vi "Item Click.vi"(4 "Menu in":refnum<class "MGI_ToolStrip.lvclass">, 5 "Event Data":cluster{"sender":refnum<k24>, "e":refnum<k24>}, 6 "Control Ref":refnum<k24>, 7 "Event Common Data":T1) -> ()   [LabVIEW 2019, in "MGI_ToolStrip.lvclass"]
uses:
  MGI_ToolStrip.lvclass
  System.Windows.Forms
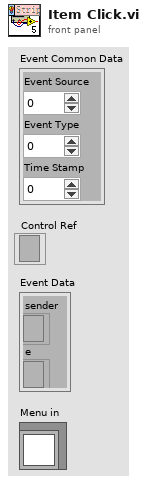
[diagram p1: front panel]
types:
  T1 = cluster{"Event Source":i32, "Event Type":u32, "Time Stamp":u32}
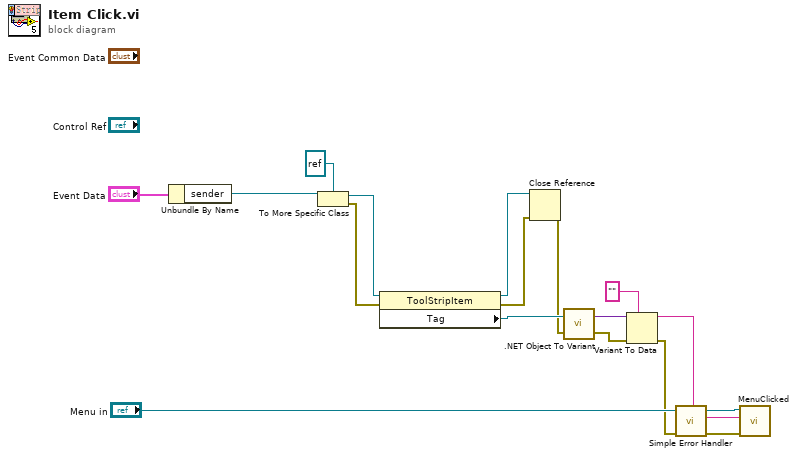
[diagram p0: block diagram]
diagram:
  n1 = Unbundle By Name("Event Data") -> ("sender"=w14:refnum<k24>)
  n2 = To More Specific Class(target class=refnum<k24> refnum ("new reference"), reference=w14) -> (specific class reference=w13:refnum<k24>, error out=w3:errorcluster)  [unwired: 1 in]
  n3 = property class="ToolStripItem"(reference=w13, error in=w3) -> (reference out=w12:refnum<k24>, error out=w11:errorcluster, "Tag"=w7:refnum<k24>)
  n4 = Close Reference(reference=w12, error in (no error)=w11) -> (error out=w2:errorcluster)
  n5 = call <vilib>:".NET Object To Variant.vi"("error in (no error)"=w2, ".NET object"=w7) -> ("error out"=w9:errorcluster, "variant"=w10:variant)
  n6 = Variant To Data(error in=w9, type="", Variant=w10) -> (data=w1:string, error out=w5:errorcluster)
  n7 = call <vilib>:"Simple Error Handler.vi"("error in (no error)"=w5) -> ("error out"=w4:errorcluster)  [unwired: 4 in, 4 out]
  n8 = call-dynamic "MenuClicked.vi"("error in (no error)"=w4, "Full Tag"=w1, "Menu in"="Menu in") -> ()  [unwired: 7 in, 2 out]
